vi "CamSnapTest.vi"() -> ()   [LabVIEW 2016]
uses:
  <vilib>/userdefined/High Color/IMAQdx.ctl
  <vilib>/vision/driver/NI_Vision_Acquisition_Software.lvlib
panel:
  out "Loop #":i32
  out "Array 2":string[](array[string])
  in  "Nsnaps":i32
  out "Array":T1[](array[plugin-control])
  out "Main":i32
  in  "Gain":dbl(slide)=4.875739644970414 scale=0.0..15.9
  in  "Get snap":bool
  in  "stop":bool
  out "Snap":T1(plugin-control)
  out "Grab":T1(plugin-control)
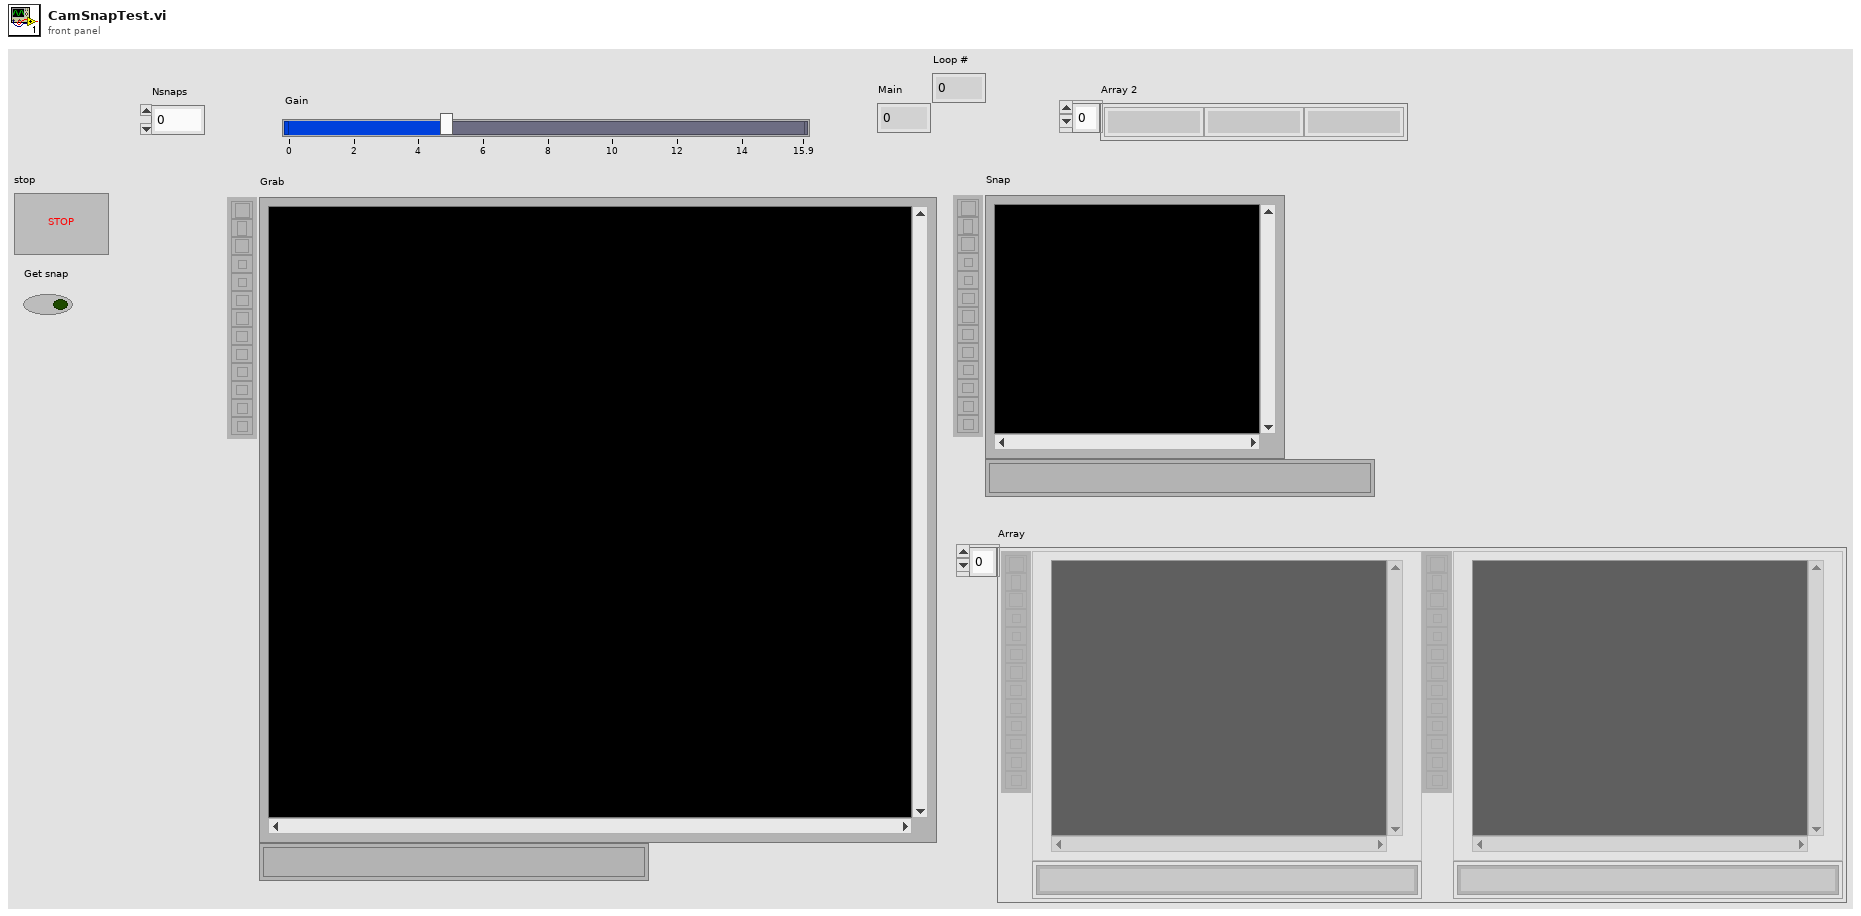
[diagram p1: front panel]
types:
  T1 = typedef "IMAQ Image.ctl" = refnum<image>
  T2 = typedef "IMAQdx.ctl" = refnum<k21>
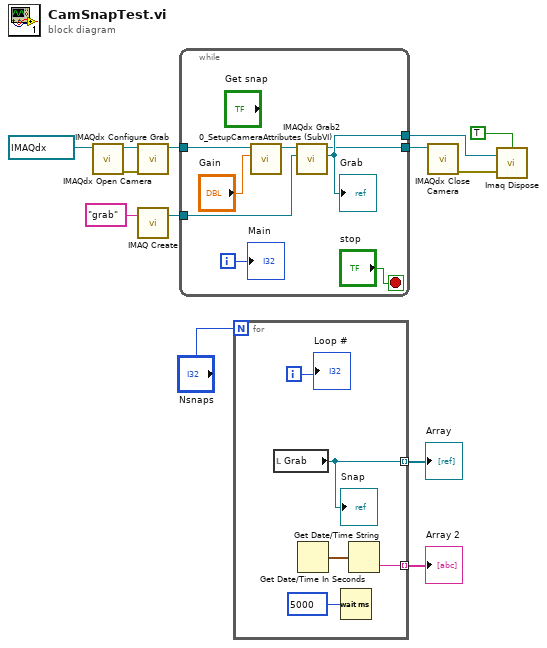
[diagram p0: block diagram]
diagram:
  n1 = call <vilib>:"IMAQdx Open Camera.vi"("Session In"=T2 "cam1") -> ("error out"=w13:errorcluster, "Session Out"=w12:T2)  [unwired: 9 in]
  n2 = call <vilib>:"IMAQdx Configure Grab.vi"("error in"=w13, "Session In"=w12) -> ("Session Out"=w5:T2)  [unwired: 8 in, 1 out]
  n3 = call "IMAQ Create"("Image Name"="grab") -> ("New Image"=w9:T1)  [unwired: 4 in, 1 out]
  n4 = while {
    tunnel: w9 -> [w21]
    tunnel: [w19] -> w8
    tunnel: [w18] -> w6
    tunnel: w5 -> [w17]
    i -> [w14]
    stop <- "stop" stop-if-true
    n5 = call "0_SetupCameraAttributes (SubVI).vi"("Gain"="Gain", "Camera session in"=w17) -> ("Camera session out"=w16:T2)  [unwired: 8 in, 1 out]
    n6 = call <vilib>:"IMAQdx Grab2.vi"("Image In"=w21, "Session In"=w16) -> ("Image Out"=w19:T1, "Session Out"=w18:T2)  [unwired: 6 in, 2 out]
    "Grab" <- w19
    "Main" <- w14
  }
  n7 = for {
    N: "Nsnaps" -> [_]
    tunnel: [w26] -> w3 mode=indexing
    tunnel: [w23] -> w1 mode=indexing
    i -> [w22]
    n8 = local read "Grab"() -> (w26:T1)
    "Snap" <- w26
    n9 = Get Date/Time In Seconds() -> (seconds since 1Jan1904=w24:timestamp)
    n10 = Wait (ms)(milliseconds to wait=u32 5000) -> ()  [unwired: 1 out]
    n11 = Get Date/Time String(seconds (now)=w24) -> (time string=w23:string)  [unwired: 2 in, 1 out]
    "Loop #" <- w22
  }
  "Array" <- w3
  "Array 2" <- w1
  n12 = call <vilib>:"IMAQdx Close Camera.vi"("Session In"=w6) -> ("error out"=w7:errorcluster)  [unwired: 10 in]
  n13 = call "Imaq Dispose"("All Images? (No)"=TRUE, "Image"=w8, "error in (no error)"=w7) -> ()  [unwired: 3 in, 1 out]
